vi "EditConfig.vi"(2 "error in":errorcluster) -> (0 "error out":errorcluster, 1 "Cancelled?":bool)   [LabVIEW 2010]
uses:
  Typedefs/AxisSpaceCfg_ArrayofAxisCfg.ctl
  Typedefs/AxisCfg_cluster.ctl
  <vilib>/Motion/FlexMotion/CustomControls/CustomControls.llb/Axis To Read.flx
  Globals/AxisSpace.vi
panel:
  in  "Export":bool
  in  "Import":bool
  in  "Cancel Button":bool
  in  "OK Button":bool
  in  "Axis Space Config":T1 {"Axis" items=["Axis 1"=1, "Axis 2"=2, "Axis 3"=3, "Axis 4"=4, "Axis 5"=5, "Axis 6"=6, "Axis 7"=7, "Axis 8"=8]}
  # "Axis 1"
  # "Axis 2"
  # "Axis 3"
  # "Axis 4"
  # "Axis 5"
  # "Axis 6"
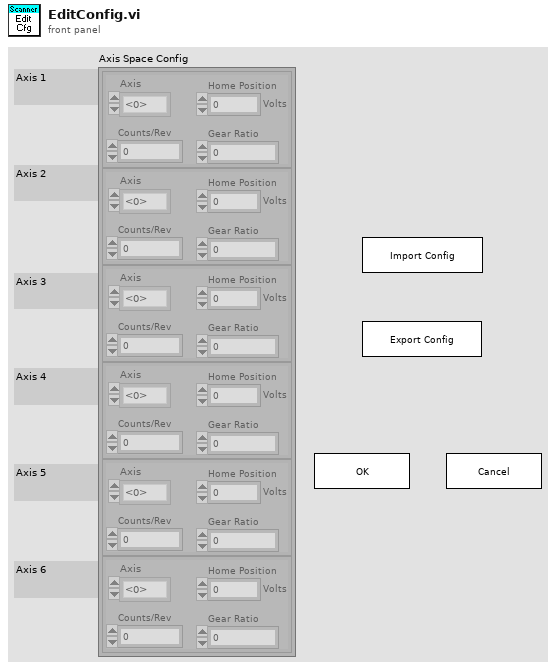
[diagram p1: front panel]
types:
  T1 = typedef "AxisSpaceCfg_ArrayofAxisCfg.ctl" = T2[]
  T2 = typedef "AxisCfg_cluster.ctl" = cluster{"Axis":T3, "Counts/Rev":dbl, "Gear Ratio":dbl, "Home Position":dbl}
  T3 = typedef "Axis To Read.flx" = u16
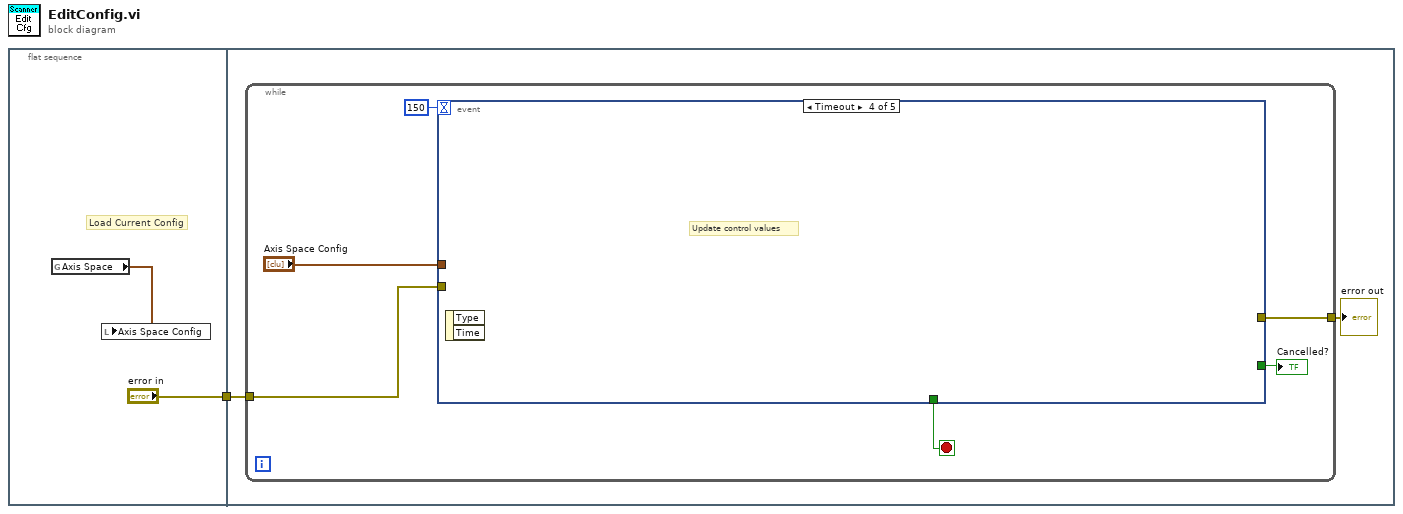
[diagram p0: block diagram]
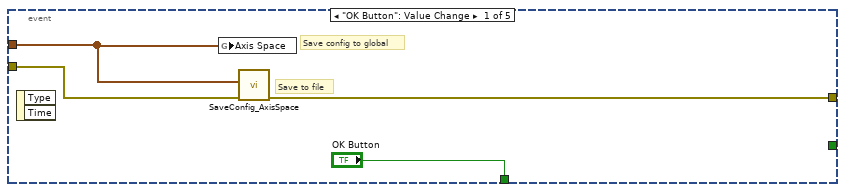
[diagram p2: hidden frame]
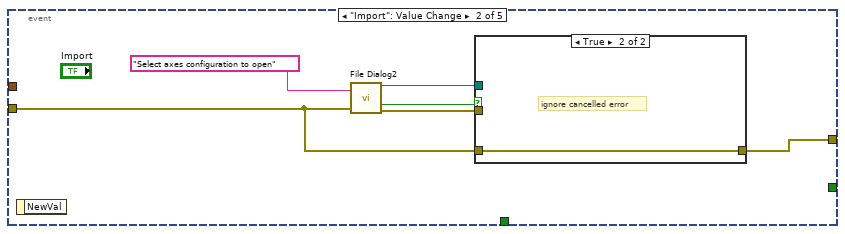
[diagram p3: hidden frame]
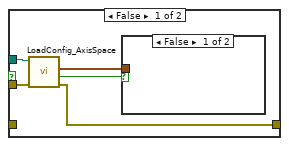
[diagram p4: hidden frame]
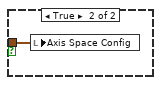
[diagram p5: hidden frame]
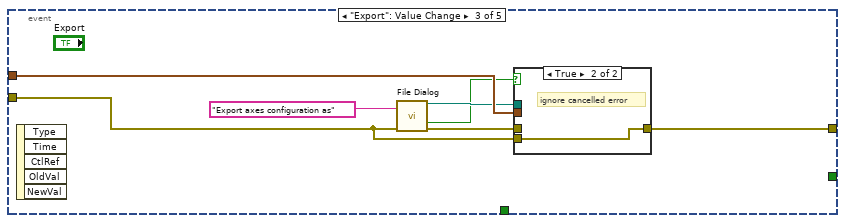
[diagram p6: hidden frame]
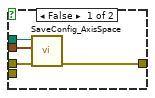
[diagram p7: hidden frame]
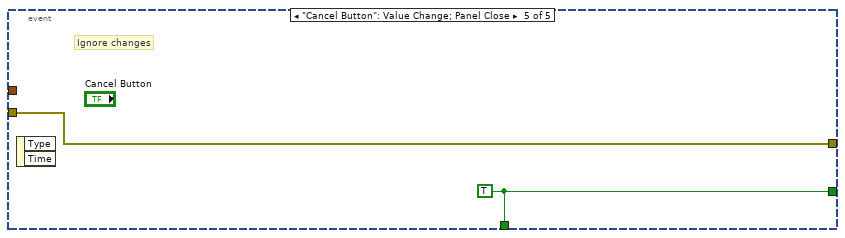
[diagram p8: hidden frame]
diagram:
  n1 = flat-sequence {
    tunnel: ["error in"] -> w1
    tunnel: w1 -> [w4]
    frame #0 {
      # "Load Current Config"
      n2 = global read "AxisSpace.vi" "Axis Space"() -> (w3:T1)
      n3 = local write "Axis Space Config"(w3) -> ()
    }
    frame #1 {
      n4 = while {
        tunnel: [w9] -> w5
        tunnel: w4 -> [w8]
        stop <- w10 stop-if-true
        n5 = event shown="[3] Timeout" {
          selector: _ -> [_ _ _ _ _]
          dyn-events: _ -> [_ _ _ _ _]
          timeout: 150 -> [_ _ _ _ _]
          tunnel: "Axis Space Config" -> [w15 _ w35 _ _]
          tunnel: ["OK Button" _ _ _ w41] -> w10
          tunnel: [w13 w21 w34 _ w42] -> w9
          tunnel: w8 -> [w12 w16 w29 _ w42]
          tunnel: [_ _ _ _ w41] -> w6
          event "OK Button": Value Change {
            # "Save to file"
            # "Save config to global"
            n6 = event-data() -> ()  [unwired: 1 in, 2 out]
            n7 = global write "AxisSpace.vi" "Axis Space"(w15) -> ()
            n8 = call "SaveConfig_AxisSpace.vi"("error in (no error)"=w12, "Axis Space Config"=w15) -> ("error out"=w13:errorcluster)  [unwired: 9 in]
          }
          event "Import": Value Change {
            n9 = event-data() -> ()  [unwired: 1 in, 1 out]
            n10 = call "File Dialog2"("prompt"="Select axes configuration to open", "error in"=w16) -> ("selected path"=w17:path, "cancelled"=w19:bool, "error out"=w18:errorcluster)  [unwired: 10 in, 1 out]
            n11 = case shown="True" w19 {
              tunnel: w18 -> [w24 _]
              tunnel: w17 -> [w23 _]
              tunnel: [w22 w28] -> w21
              tunnel: w16 -> [_ w28]
              frame False {
                n12 = call "LoadConfig_AxisSpace.vi"("error in (no error)"=w24, "Path (.AxisSpace.cfg)"=w23) -> ("error out"=w22:errorcluster, "file or folder exists?"=w26:bool, "Axis Space"=w25:T1)  [unwired: 7 in]
                n13 = case shown="False" w26 {
                  tunnel: w25 -> [_ w27]
                  frame False {
                  }
                  frame True {
                    n14 = local write "Axis Space Config"(w27) -> ()
                  }
                }
              }
              frame True {
                # "ignore cancelled error"
              }
            }
          }
          event "Export": Value Change {
            n15 = event-data() -> ()  [unwired: 1 in, 5 out]
            n16 = call "File Dialog"("prompt"="Export axes configuration as", "error in"=w29) -> ("selected path"=w33:path, "cancelled"=w30:bool, "error out"=w32:errorcluster)  [unwired: 10 in, 1 out]
            n17 = case shown="True" w30 {
              tunnel: w33 -> [w39 _]
              tunnel: w35 -> [w38 _]
              tunnel: w32 -> [w37 _]
              tunnel: [w36 w40] -> w34
              tunnel: w29 -> [_ w40]
              frame False {
                n18 = call "SaveConfig_AxisSpace.vi"("error in (no error)"=w37, "Axis Space Config"=w38, "Path (.AxisSpace.cfg)"=w39) -> ("error out"=w36:errorcluster)  [unwired: 8 in]
              }
              frame True {
                # "ignore cancelled error"
              }
            }
          }
          event Timeout {
            # "Update control values"
            n19 = event-data() -> ()  [unwired: 1 in, 2 out]
          }
          event "Cancel Button": Value Change; Panel Close {
            w41 = TRUE ("x")
            # "Ignore changes"
            n20 = event-data() -> ()  [unwired: 1 in, 2 out]
          }
        }
        "Cancelled?" <- w6
      }
      "error out" <- w5
    }
  }
